vi "Plot Model.vi"(8 "error in (no error)":errorcluster, 10 "Input onfiguration":T1 {"Gnormal" format="%#_6p"; "Model parameters gap 2"."Delta 1" step=0.001 format="%#_6peV"; "Model parameters gap 2"."Resolution" format="%#_6peV"; "Model parameters gap 2"."Integration range" format="%#_6peV"; "Model parameters gap 2"."T" format="%#_6pK"; "Model parameters gap 2"."Delta 2" step=0.001 format="%#_6peV"; "Model parameters gap 2"."Gama" step=0.001 format="%#_6peV"; "Offset" scale=0.0..0.1; "Scale" scale=0.0..0.03; "Model parameters gap 1"."Delta 1" step=0.001 format="%#_6peV"; "Model parameters gap 1"."Resolution" format="%#_6peV"; "Model parameters gap 1"."Integration range" format="%#_6peV"; "Model parameters gap 1"."T" format="%#_6pK"; "Model parameters gap 1"."Delta 2" step=0.001 format="%#_6peV"; "Model parameters gap 1"."Gama" step=0.001 format="%#_6peV"; "Resistance in series" scale=0.0..80.0}, 11 "dIdV State in":refnum<class "Point Contact Model.lvclass">) -> (0 "error out":errorcluster, 3 "dIdV State out":refnum<class "Point Contact Model.lvclass">)   [LabVIEW 2021, in "Point Contact Model.lvclass"]
uses:
  Point Contact Model.lvclass
  Controls/PCS Config.ctl
  Parameters.ctl
  Point Contact Model.lvclass/Point Contact Model.ctl
panel:
  # "<="
  # "<="
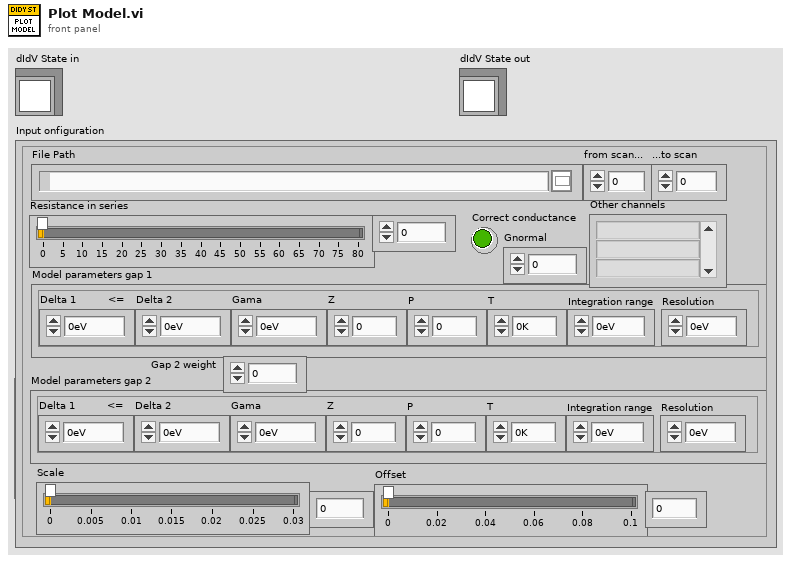
[diagram p1: front panel]
types:
  T1 = typedef "PCS Config.ctl" = cluster{"File Path":path, "from scan...":i32, "...to scan":i32, "Resistance in series":dbl, "Correct conductance ":bool, "Model parameters gap 1":T2, "Scale":dbl, "Offset":dbl, "Other channels":string[], "Model parameters gap 2":T2, "Gap 2 weight":dbl, "Gnormal":dbl}
  T2 = typedef "Parameters.ctl" = cluster{"Delta 1":dbl, "Delta 2":dbl, "Gama":dbl, "Z":dbl, "P":dbl, "T":dbl, "Integration range":dbl, "Resolution":dbl}
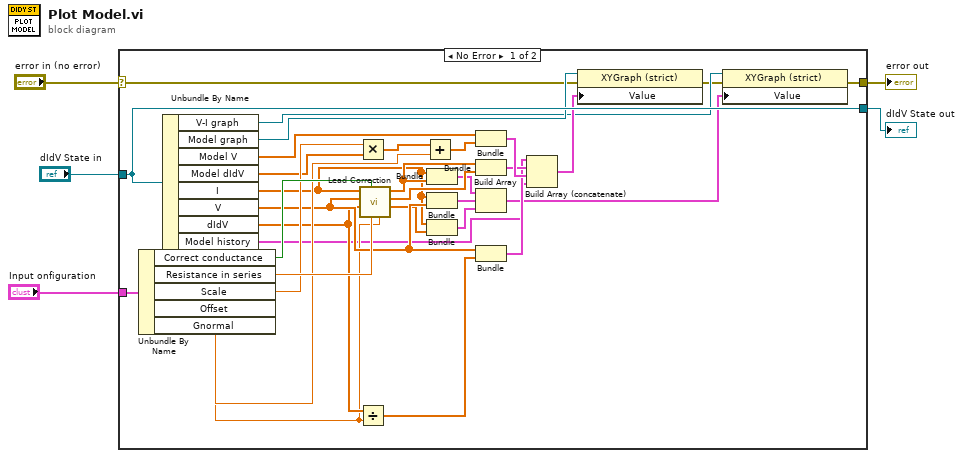
[diagram p0: block diagram]
diagram:
  n1 = case shown="No Error" "error in (no error)" {
    selector: "error in (no error)" -> [w28 w39]
    tunnel: [w18 w39] -> w4
    tunnel: [w35 w38] -> w2
    tunnel: "dIdV State in" -> [w35 w38]
    tunnel: "Input onfiguration" -> [w34 _]
    frame No Error {
      n2 = Unbundle By Name(w34) -> ("Correct conductance"=w36:bool, "Resistance in series"=w37:dbl, "Scale"=w26:dbl, "Offset"=w24:dbl, "Gnormal"=w8:dbl)
      n3 = Unbundle By Name(w35) -> ("V-I graph"=w20:refnum<vi>, "Model graph"=w30:refnum<vi>, "Model V"=w32:dbl[], "Model dIdV"=w25:dbl[], "I"=w12:dbl[], "V"=w14:dbl[], "dIdV"=w9:dbl[], "Model history"=w6:cluster{"Model V":dbl[], "Model dIdV":dbl[]}[])
      n4 = Multiply(x=w26, y=w25) -> (x*y=w27:dbl[])
      n5 = Divide(x=w9, y=w8) -> (x/y=w7:dbl[])
      n6 = call "Lead Correction.vi"("Gnormal"=w8, "Resistance in series"=w37, "Correct conductance"=w36, "dIdV"=w9, "V"=w14, "I"=w12) -> ("V correction"=w11:dbl[], "dIdV out"=w33:dbl[], "V out"=w16:dbl[])  [unwired: 2 in, 1 out]
      n7 = Add(x=w27, y=w24) -> (x+y=w23:dbl[])
      n8 = Bundle("I"=w12, "V out"=w16) -> (w15:cluster{"I":dbl[], "V out":dbl[]})  [unwired: 1 in]
      n9 = Bundle("I"=w12, "V"=w14) -> (w13:cluster{"I":dbl[], "V":dbl[]})  [unwired: 1 in]
      n10 = Bundle("I"=w12, "V correction"=w11) -> (w10:cluster{"I":dbl[], "V correction":dbl[]})  [unwired: 1 in]
      n11 = Bundle("Model V"=w32, w23) -> (w31:cluster{"Model V":dbl[], dbl[]})  [unwired: 1 in]
      n12 = Bundle("V out"=w16, "dIdV out"=w33) -> (w22:cluster{"V out":dbl[], "dIdV out":dbl[]})  [unwired: 1 in]
      n13 = Build Array(w15, w13, w10) -> (w17:cluster{"I":dbl[], "V correction":dbl[]}[])
      n14 = Bundle("V"=w14, w7) -> (w21:cluster{"V":dbl[], dbl[]})  [unwired: 1 in]
      n15 = Build Array (concatenate)(w21, w22, w31, w6) -> (w29:cluster{"Model V":dbl[], "Model dIdV":dbl[]}[])
      n16 = property class="XYGraph (strict)"(reference=w30, error in=w28, "Value"=w29) -> (error out=w19:errorcluster)  [unwired: 1 out]
      n17 = property class="XYGraph (strict)"(reference=w20, error in=w19, "Value"=w17) -> (error out=w18:errorcluster)  [unwired: 1 out]
    }
    frame Error {
    }
  }
  "error out" <- w4
  "dIdV State out" <- w2
